vi "QuickDrop Insert String into Array.vi"(6 "Secondary String":string, 9 "Secondary Array in":string[](array[string]), 10 "Primary String":string, 11 "Primary Array in":string[](array[string])) -> (1 "Secondary Array out":string[](array[string]), 3 "Primary Array out":string[](array[string]))   [LabVIEW 2016]
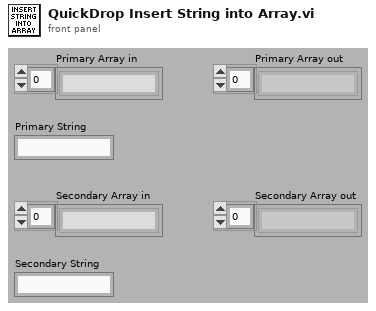
[diagram p1: front panel]
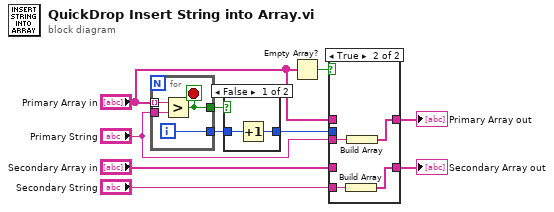
[diagram p0: block diagram]
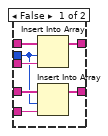
[diagram p2: hidden frame]
diagram:
  n1 = for {
    tunnel: "Primary Array in" -> [w13] mode=indexing
    tunnel: "Primary String" -> [w12]
    tunnel: [w14] -> w10
    tunnel: [w11] -> w8
    i -> [w14]
    stop <- w11 stop-if-true
    n2 = Greater?(x=w13, y=w12) -> (0:w11:bool)
  }
  n3 = case shown="False" w8 {
    tunnel: [w16 w17] -> w9
    tunnel: w10 -> [w15 w17]
    frame False {
      n4 = Increment(x=w15) -> (x+1=w16:i32)
    }
    frame True {
    }
  }
  n5 = Empty Array?(array="Primary Array in") -> (empty?=w4:bool)
  n6 = case shown="True" w4 {
    tunnel: w9 -> [w19 _]
    tunnel: "Primary String" -> [w24 w28]
    tunnel: [w23 w27] -> w6
    tunnel: "Primary Array in" -> [w22 _]
    tunnel: [w21 w25] -> w3
    tunnel: "Secondary Array in" -> [w20 _]
    tunnel: "Secondary String" -> [w18 w26]
    frame False {
      n7 = Insert Into Array(array=w22, index=w19, new element=w24) -> (w23:string[])
      n8 = Insert Into Array(array=w20, index=w19, new element=w18) -> (w21:string[])
    }
    frame True {
      n9 = Build Array(w26) -> (w25:string[])
      n10 = Build Array(w28) -> (w27:string[])
    }
  }
  "Primary Array out" <- w6
  "Secondary Array out" <- w3
